vi "Get Subsystem by Name.vi"(8 "error in (no error)":errorcluster, 10 "Name":string) -> (0 "error out":errorcluster, 1 "found":bool, 2 "Subsystem":refnum<class "SMO.lvclass">)   [LabVIEW 2021, in "smo.lvlib" / "Registry-SMO.lvclass"]
uses:
  Registry-SMO.lvclass
  Registry-SMO.lvclass/Registry-SMO.ctl
  SMO/SMO.lvclass
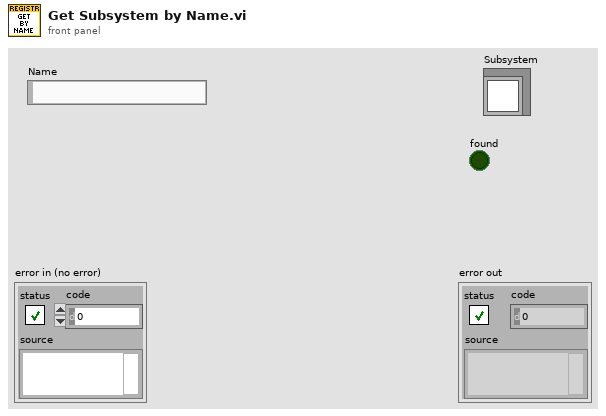
[diagram p1: front panel]
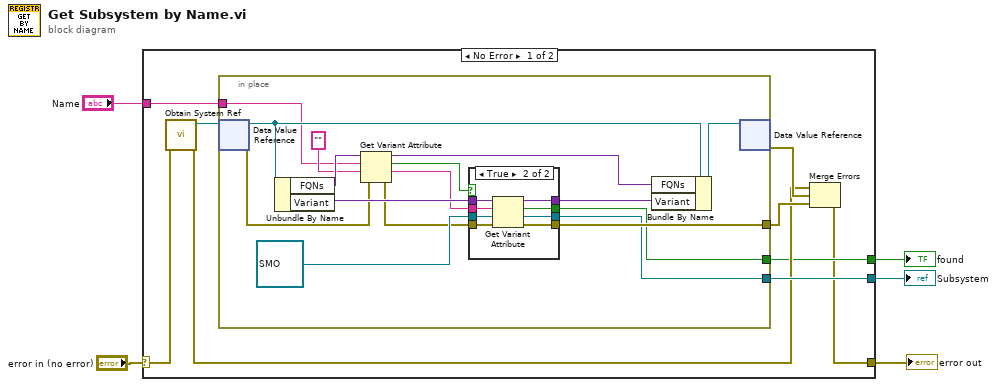
[diagram p0: block diagram]
diagram:
  n1 = case shown="No Error" "error in (no error)" {
    selector: "error in (no error)" -> [w10 w42]
    tunnel: [w6 w42] -> w4
    tunnel: [w12 _] -> w3
    tunnel: "Name" -> [w8 _]
    tunnel: [w7 _] -> w1
    frame No Error {
      n2 = call "Obtain System Ref.vi"("error in (no error)"=w10) -> ("error out"=w9:errorcluster, "JKI SMO System"=w11:refnum<data-value>)  [unwired: 9 in]
      n3 = in-place {
        in-place-border: [w26] -> w13
        in-place-border: [w24] -> w12
        in-place-border: w8 -> [w20]
        in-place-border: [w23] -> w7
        n4 = in-place-dvr #1(w11) -> (w30:refnum<class "Registry-SMO.lvclass">, w18:errorcluster)
        n5 = Unbundle By Name(w30) -> ("FQNs"=w22:variant, "Variant"=w28:variant)
        n6 = Get Variant Attribute(Variant=w22, name=w20, default value (empty Variant)="", error in=w18) -> (duplicate Variant=w16:variant, found=w15:bool, value=w19:string, error out=w17:errorcluster)
        n7 = case shown="True" w15 {
          tunnel: w28 -> [w33 w41]
          tunnel: [w33 w40] -> w27
          tunnel: [w31 w39] -> w26
          tunnel: refnum<class "SMO.lvclass"> refnum ("JKI SMO.lvclass") -> [w32 w38]
          tunnel: [w32 w37] -> w24
          tunnel: [_ w36] -> w23
          tunnel: w19 -> [_ w35]
          tunnel: w17 -> [w31 w34]
          frame False {
          }
          frame True {
            n8 = Get Variant Attribute(Variant=w41, name=w35, default value (empty Variant)=w38, error in=w34) -> (duplicate Variant=w40:variant, found=w36:bool, value=w37:refnum<class "SMO.lvclass">, error out=w39:errorcluster)
          }
        }
        n9 = Bundle By Name(cluster=w30, "FQNs"=w16, "Variant"=w27) -> (w29:refnum<class "Registry-SMO.lvclass">)
        n10 = in-place-dvr #1(w29) -> (w14:errorcluster)  [unwired: 1 out]
      }
      n11 = Merge Errors(w9, w14, w13) -> (w6:errorcluster)
    }
    frame Error {
    }
  }
  "error out" <- w4
  "Subsystem" <- w3
  "found" <- w1
